vi "Encoder Read.vi"(8 "error in (no error)":errorcluster, 11 "Task In":T1) -> (0 "error out":errorcluster, 2 "Posição":i32, 3 "Task Out":T1)   [LabVIEW 2018]
uses:
  <vilib>/DAQmx/write.llb/DAQmx Write (Digital Bool 1Line 1Point).vi
  <vilib>/DAQmx/read.llb/DAQmx Read (Analog 1D DBL 1Chan NSamp).vi
  <vilib>/DAQmx/configure/trigger.llb/DAQmx Start Trigger (Digital Edge).vi
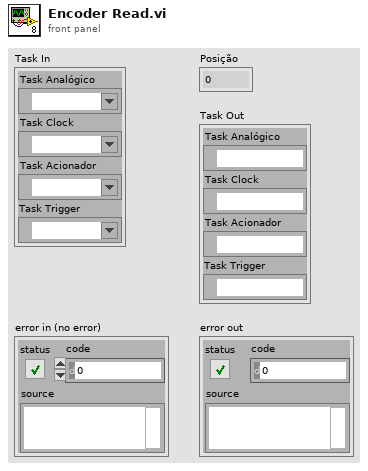
[diagram p1: front panel]
types:
  T1 = cluster{"Task Analógico":refnum<k21>, "Task Clock":refnum<k21>, "Task Acionador":refnum<k21>, "Task Trigger":tag}
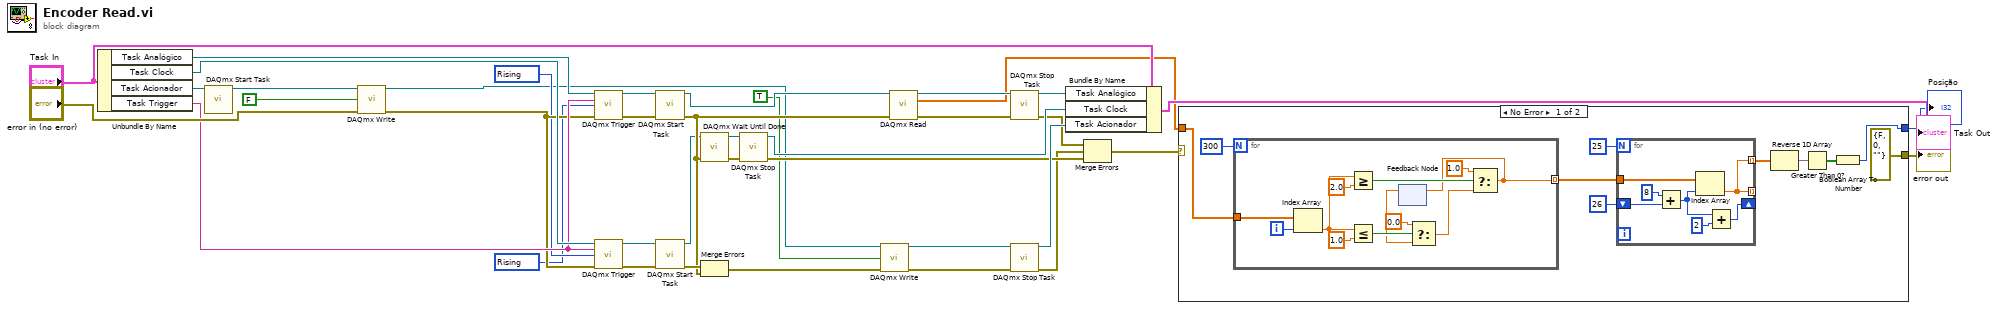
[diagram p0: block diagram]
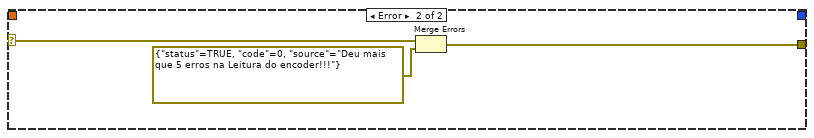
[diagram p2: hidden frame]
diagram:
  w15 = 10280 items=["Rising"=10280, "Falling"=10171] ("Edge")
  w12 = 10280 items=["Rising"=10280, "Falling"=10171] ("Edge")
  n1 = Unbundle By Name("Task In") -> ("Task Analógico"=w31:refnum<k21>, "Task Clock"=w33:refnum<k21>, "Task Acionador"=w32:refnum<k21>, "Task Trigger"=w30:tag)
  n2 = call <vilib>:"DAQmx Start Task.vi"("task/channels in"=w32) -> ("task out"=w7:refnum<k21>)  [unwired: 13 in, 1 out]
  n3 = call-poly <vilib>:"DAQmx Write.vi"("task/channels in"=w7, "data"=FALSE, "error in"="error in (no error)") -> ("task out"=w4:refnum<k21>, "error out"=w18:errorcluster)  [unwired: 10 in, 1 out]
  n4 = call-poly <vilib>:"DAQmx Trigger.vi"("task/channels in"=w31, "source"=w30, "edge"=w12, "error in"=w18) -> ("task out"=w16:refnum<k21>, "error out"=w19:errorcluster)  [unwired: 10 in]
  n5 = call-poly <vilib>:"DAQmx Trigger.vi"("task/channels in"=w33, "source"=w30, "edge"=w15, "error in"=w18) -> ("task out"=w14:refnum<k21>, "error out"=w17:errorcluster)  [unwired: 10 in]
  n6 = call <vilib>:"DAQmx Start Task.vi"("task/channels in"=w16, "error in"=w19) -> ("task out"=w8:refnum<k21>, "error out"=w20:errorcluster)  [unwired: 12 in]
  n7 = call <vilib>:"DAQmx Start Task.vi"("task/channels in"=w14, "error in"=w17) -> ("task out"=w13:refnum<k21>, "error out"=w21:errorcluster)  [unwired: 12 in]
  n8 = call <vilib>:"DAQmx Wait Until Done.vi"("task/channels in"=w13, "error in"=w20) -> ("task out"=w10:refnum<k21>, "error out"=w23:errorcluster)  [unwired: 12 in]
  n9 = Merge Errors(w21, w20) -> (w22:errorcluster)
  n10 = call <vilib>:"DAQmx Stop Task.vi"("task/channels in"=w10, "error in"=w23) -> ("task out"=w36:refnum<k21>, "error out"=w28:errorcluster)  [unwired: 12 in]
  n11 = call-poly <vilib>:"DAQmx Write.vi"("task/channels in"=w4, "data"=TRUE ("stop (T)"), "error in"=w22) -> ("task out"=w9:refnum<k21>, "error out"=w24:errorcluster)  [unwired: 10 in, 1 out]
  n12 = call-poly <vilib>:"DAQmx Read.vi"("task/channels in"=w8, "error in"=w20) -> ("task out"=w11:refnum<k21>, "data"=w2:dbl[], "error out"=w25:errorcluster)  [unwired: 11 in]
  n13 = call <vilib>:"DAQmx Stop Task.vi"("task/channels in"=w11, "error in"=w25) -> ("task out"=w35:refnum<k21>, "error out"=w26:errorcluster)  [unwired: 12 in]
  n14 = call <vilib>:"DAQmx Stop Task.vi"("task/channels in"=w9, "error in"=w24) -> ("task out"=w37:refnum<k21>, "error out"=w27:errorcluster)  [unwired: 12 in]
  n15 = Bundle By Name(cluster="Task In", "Task Analógico"=w35, "Task Clock"=w36, "Task Acionador"=w37) -> (→"Task Out":T1)
  n16 = Merge Errors(w26, w27, w28) -> (w29:errorcluster)
  n17 = case shown="No Error" w29 {
    selector: w29 -> [_ w71]
    tunnel: [errorcluster {"status"=FALSE, "code"=0, "source"=""} ("error IO") w70] -> w1
    tunnel: w2 -> [w42 _]
    tunnel: [w40 _] -> w6
    frame No Error {
      n18 = for {
        N: 300 -> [_]
        tunnel: w42 -> [w68]
        tunnel: [w59] -> w46 mode=indexing
        i -> [w67]
        n19 = Index Array(array=w68, index=w67) -> (element=w57:dbl)
        n20 = Greater Or Equal?(x=w57, y=2.0) -> (x >= y?=w66:bool)
        n21 = Less Or Equal?(x=w57, y=1.0) -> (x <= y?=w64:bool)
        n22 = feedback #1() -> (w58:dbl)  [unwired: 1 in]
        n23 = Select(t=0.0, s=w64, f=w58) -> (s? t:f=w63:dbl)
        n24 = Select(t=1.0, s=w66, f=w63) -> (s? t:f=w59:dbl)
        n25 = feedback-in #1(w59) -> ()
      }
      n26 = for {
        N: 25 -> [_]
        tunnel: w46 -> [w55]
        tunnel: [w50] -> w41 mode=indexing
        shift-right: [w53] -> _
        shift-left: 26 -> [w52]
        tunnel: [w50] -> _ mode=indexing
        n27 = Add(x=8, y=w52) -> (x+y=w51:i32)
        n28 = Index Array(array=w55, index=w51) -> (element=w50:dbl)
        n29 = Add(x=w51, y=2) -> (x+y=w53:i32)
      }
      n30 = Reverse 1D Array(array=w41) -> (reversed array=w44:dbl[])
      n31 = Greater Than 0?(x=w44) -> (x > 0?=w45:bool[])
      n32 = Boolean Array To Number(Boolean array=w45) -> (number=w40:i32)
    }
    frame Error {
      n33 = Merge Errors(w71, errorcluster {"status"=TRUE, "code"=0, "source"="Deu mais que 5 erros na Leitura do encoder!!!"} ("error in")) -> (w70:errorcluster)
    }
  }
  "Posição" <- w6
  "error out" <- w1
